vi "2_key_char_check.vi"(8 "value 1":dbl, 9 "keys pressed[1]":dbl, 10 "value 0":dbl, 11 "keys pressed[0]":dbl) -> (2 "control":bool)   [LabVIEW 2011]
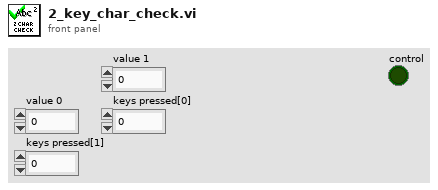
[diagram p1: front panel]
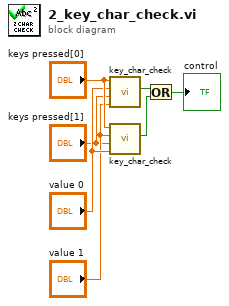
[diagram p0: block diagram]
diagram:
  n1 = call "key_char_check.vi"("key value[1]"="value 1", "keys pressed[1]"="keys pressed[1]", "key value[0]"="value 0", "keys pressed[0]"="keys pressed[0]") -> ("control"=w7:bool)  [unwired: 7 in]
  n2 = call "key_char_check.vi"("key value[1]"="value 0", "keys pressed[1]"="keys pressed[1]", "key value[0]"="value 1", "keys pressed[0]"="keys pressed[0]") -> ("control"=w6:bool)  [unwired: 7 in]
  n3 = Or(x=w7, y=w6) -> (x .or. y?=→"control":bool)
